vi "SetZeroPosition.vi"(4 "error in (no error)":errorcluster, 5 "Motor":i32, 6 "DeviceKey In":string, 7 "CmdLib In":refnum<k24>) -> (0 "error out":errorcluster, 2 "DeviceKey Out":string, 3 "CmdLib Out":refnum<k24>)   [LabVIEW 2014]
uses:
  C:/Users/Hexagon/Documents/git/DevPyController/labview/cesium_controller/PicoMotor/NewFocus8742/CmdLib.dll
  CmdLib.dll
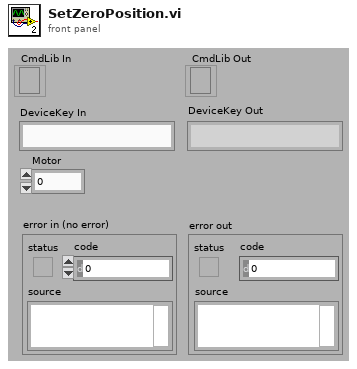
[diagram p1: front panel]
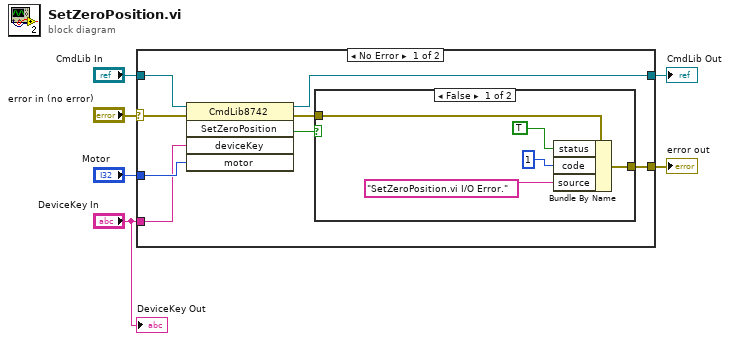
[diagram p0: block diagram]
diagram:
  n1 = case shown="No Error" "error in (no error)" {
    selector: "error in (no error)" -> [w10 w21]
    tunnel: "CmdLib In" -> [w14 w22]
    tunnel: [w13 w22] -> w5
    tunnel: "Motor" -> [w12 _]
    tunnel: "DeviceKey In" -> [w11 _]
    tunnel: [w7 w21] -> w2
    frame No Error {
      n2 = invoke class="CmdLib8742" method="SetZeroPosition"(reference=w14, error in=w10, "deviceKey"=w11, "motor"=w12) -> (reference out=w13:refnum<k24>, error out=w8:errorcluster, "SetZeroPosition"=w9:bool)  [unwired: 1 in, 2 out]
      n3 = case shown="False" w9 {
        tunnel: w8 -> [w19 w20]
        tunnel: [w18 w20] -> w7
        frame False {
          n4 = Bundle By Name(cluster=w19, "status"=TRUE, "code"=1, "source"="SetZeroPosition.vi I/O Error.") -> (w18:errorcluster)
        }
        frame True {
        }
      }
    }
    frame Error {
    }
  }
  "error out" <- w2
  "CmdLib Out" <- w5
  "DeviceKey Out" <- "DeviceKey In"
